vi "Nearest Even.vi"(1 "digit":i8) -> (0 "Rounded to even":i8)   [LabVIEW 2025]
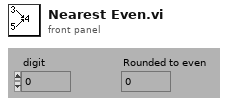
[diagram p1: front panel]
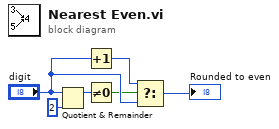
[diagram p0: block diagram]
diagram:
  n1 = Quotient & Remainder(x="digit", y=i8 2) -> (x-y*floor(x/y)=w3:i8)  [unwired: 1 out]
  n2 = Increment(x="digit") -> (x+1=w1:i8)
  n3 = Not Equal To 0?(x=w3) -> (x != 0?=w2:bool)
  n4 = Select(t=w1, s=w2, f="digit") -> (s? t:f=→"Rounded to even":i8)
